vi "Read Attributes.vi"(11 "Return VF Device UID Msg":refnum<class "Return VF Device UID Msg.lvclass">) -> (2 "Payload":cluster{"DeviceID":u64})   [LabVIEW 2016, in "Optimization Framework.lvlib" / "Return VF Device UID Msg.lvclass"]
uses:
  Return VF Device UID Msg.lvclass
  Return VF Device UID Msg.lvclass/Return VF Device UID Msg.ctl
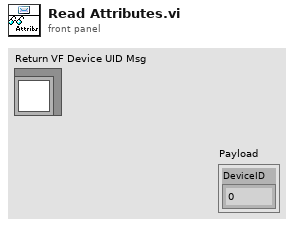
[diagram p1: front panel]
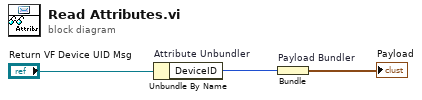
[diagram p0: block diagram]
diagram:
  n1 = Unbundle By Name "Attribute Unbundler"("Return VF Device UID Msg") -> ("DeviceID"=w1:u64)
  n2 = Bundle "Payload Bundler"("DeviceID"=w1) -> (→"Payload":cluster{"DeviceID":u64})  [unwired: 1 in]
